vi "Shortest Distance Absolute.vi"(10 "current":dbl(knob) scale=0.0..360.0, 11 "target":dbl(knob) scale=0.0..360.0) -> (3 "shortest angle":dbl)   [LabVIEW 2014]
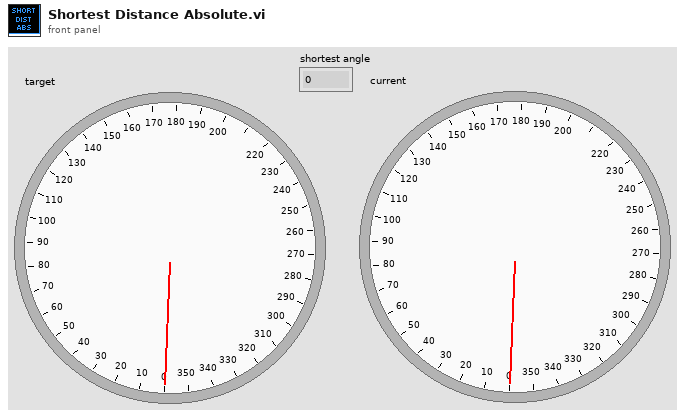
[diagram p1: front panel]
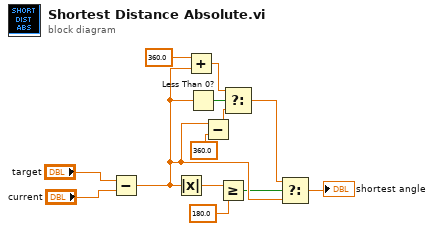
[diagram p0: block diagram]
diagram:
  n1 = Subtract(x="target", y="current") -> (x-y=w13:dbl)
  n2 = Absolute Value(x=w13) -> (abs(x)=w4:dbl)
  n3 = Add(x=360.0, y=w13) -> (x+y=w10:dbl)
  n4 = Less Than 0?(x=w13) -> (x < 0?=w8:bool)
  n5 = Subtract(x=w13, y=360.0 ("x")) -> (x-y=w9:dbl)
  n6 = Greater Or Equal?(x=w4, y=180.0) -> (x >= y?=w6:bool)
  n7 = Select(t=w10, s=w8, f=w9) -> (s? t:f=w7:dbl)
  n8 = Select(t=w7, s=w6, f=w13) -> (s? t:f=→"shortest angle":dbl)
